vi "Create.vi"(5 "String Starts With in":refnum<class "String Starts With.lvclass">, 8 "error in (no error)":errorcluster, 11 "Prefix":string) -> (0 "error out":errorcluster, 3 "String Starts With":refnum<class "String Starts With.lvclass">)   [LabVIEW 2017, in "Transparent Assertions.lvlib" / "String Starts With.lvclass"]
uses:
  String Starts With.lvclass
  String Starts With.lvclass/String Starts With.ctl
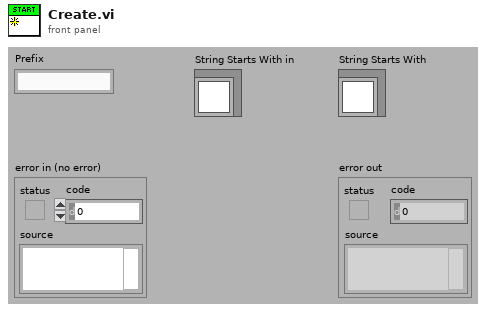
[diagram p1: front panel]
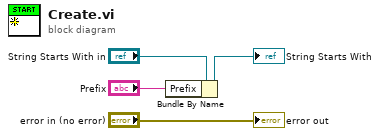
[diagram p0: block diagram]
diagram:
  n1 = Bundle By Name(cluster="String Starts With in", "Prefix"="Prefix") -> (→"String Starts With":refnum<class "String Starts With.lvclass">)
  "error out" <- "error in (no error)"
